vi "algo.get.state.vi"(11 "algo.data.in":T1={"next.state"=enum."Wait.for.Command", "saved.state"=enum."Wait.for.Command", "scratch"={"i"=0, "n"=0, "start.addr"=0, "first.call?"=FALSE, "j"=0, "o"=0, "k"=0, "p"=0, "just.write"=FALSE, "orderId "=0, "dir"=0}, "mode"=enum."Get.Symbol", "cmd.mem.watchlist"={"read.request"=FALSE, "read.addr"=0, "read.ready"=FALSE, "val.watchlist.read"={"symbol"=0, "buy.start.addr"=0, "buy.size"=0, "buy.slots"=0, "sell.start.addr"=0, "sell.size"=0, "sell.slots"=0, "min.ask"=0, "max.bid"=0}, "write.request"=FALSE, "write.addr"=0, "val.watchlist.write"={"symbol"=0, "buy.start.addr"=0, "buy.size"=0, "buy.slots"=0, "sell.start.addr"=0, "sell.size"=0, "sell.slots"=0, "min.ask"=0, "max.bid"=0}}, "cmd.mem.orders"={"read.addr"=0, "read.request"=FALSE, "read.ready"=FALSE, "write.addr"=0, "write.request"=FALSE, "read.data"={"OrderId"=0, "Price"=0, "Quantity"=0}, "write.data"={"OrderId"=0, "Price"=0, "Quantity"=0}}, "cmd.state"={"write.to.state"=FALSE, "val.state"=[0, 0, 0, 0]}, "cmd.debug"={"write.to.debug"=FALSE, "val.debug"=[0, 0]}, "stats"={"min.ask"=0, "max.bid"=0, "price"=0, "quantity"=0, "execution"=FALSE}, "orderbook.command"={"type"=enum."AddOrder", "side"=0, "orderId "=0, "quantity"=0, "symbol"=0, "price"=0, "executed.qty"=0, "canceled.qty"=0, "remaining.qty"=0, "seconds"=0, "nanoseconds"=0, "Add"=FALSE, "Edit"=FALSE, "Remove"=FALSE}, "time"={"last"=0, "since"=0}, "watchlist.size"=0, "active.watchlist"={"item"={"symbol"=0, "buy.start.addr"=0, "buy.size"=0, "buy.slots"=0, "sell.start.addr"=0, "sell.size"=0, "sell.slots"=0, "min.ask"=0, "max.bid"=0}, "index"=0}, "active.order"={"buy"=FALSE, "sell"=FALSE, "addr"=0, "size"=0, "slots"=0, "index"=0}} {"active.watchlist"."item"."symbol" format="%.0x"; "cmd.mem.orders"."write.data"."OrderId" format="%.0x"; "cmd.mem.orders"."read.data"."OrderId" format="%.0x"; "cmd.mem.watchlist"."val.watchlist.write"."symbol" format="%.0x"; "cmd.mem.watchlist"."val.watchlist.read"."symbol" format="%.0x"}) -> (3 "algo.data.out":T1={"next.state"=enum."Wait.for.Command", "saved.state"=enum."Wait.for.Command", "scratch"={"i"=0, "n"=0, "start.addr"=0, "first.call?"=FALSE, "j"=0, "o"=0, "k"=0, "p"=0, "just.write"=FALSE, "orderId "=0, "dir"=0}, "mode"=enum."Get.Symbol", "cmd.mem.watchlist"={"read.request"=FALSE, "read.addr"=0, "read.ready"=FALSE, "val.watchlist.read"={"symbol"=0, "buy.start.addr"=0, "buy.size"=0, "buy.slots"=0, "sell.start.addr"=0, "sell.size"=0, "sell.slots"=0, "min.ask"=0, "max.bid"=0}, "write.request"=FALSE, "write.addr"=0, "val.watchlist.write"={"symbol"=0, "buy.start.addr"=0, "buy.size"=0, "buy.slots"=0, "sell.start.addr"=0, "sell.size"=0, "sell.slots"=0, "min.ask"=0, "max.bid"=0}}, "cmd.mem.orders"={"read.addr"=0, "read.request"=FALSE, "read.ready"=FALSE, "write.addr"=0, "write.request"=FALSE, "read.data"={"OrderId"=0, "Price"=0, "Quantity"=0}, "write.data"={"OrderId"=0, "Price"=0, "Quantity"=0}}, "cmd.state"={"write.to.state"=FALSE, "val.state"=[0, 0, 0, 0]}, "cmd.debug"={"write.to.debug"=FALSE, "val.debug"=[0, 0]}, "stats"={"min.ask"=0, "max.bid"=0, "price"=0, "quantity"=0, "execution"=FALSE}, "orderbook.command"={"type"=enum."AddOrder", "side"=0, "orderId "=0, "quantity"=0, "symbol"=0, "price"=0, "executed.qty"=0, "canceled.qty"=0, "remaining.qty"=0, "seconds"=0, "nanoseconds"=0, "Add"=FALSE, "Edit"=FALSE, "Remove"=FALSE}, "time"={"last"=0, "since"=0}, "watchlist.size"=0, "active.watchlist"={"item"={"symbol"=0, "buy.start.addr"=0, "buy.size"=0, "buy.slots"=0, "sell.start.addr"=0, "sell.size"=0, "sell.slots"=0, "min.ask"=0, "max.bid"=0}, "index"=0}, "active.order"={"buy"=FALSE, "sell"=FALSE, "addr"=0, "size"=0, "slots"=0, "index"=0}} {"active.watchlist"."item"."symbol" format="%.0x"; "cmd.mem.orders"."write.data"."OrderId" format="%.0x"; "cmd.mem.orders"."read.data"."OrderId" format="%.0x"; "cmd.mem.watchlist"."val.watchlist.write"."symbol" format="%.0x"; "cmd.mem.watchlist"."val.watchlist.read"."symbol" format="%.0x"})   [LabVIEW 2020]
uses:
  types/algo.mode.ctl
  types/algo.states.ctl
  types/algo.scratch.ctl
  types/algo.val.watchlist.ctl
  types/algo.cmd.mem.watchlist.ctl
  types/algo.cmd.mem.orders.ctl
  types/algo.val.state.ctl
  types/algo.cmd.state.ctl
  types/algo.val.debug.ctl
  types/algo.cmd.debug.ctl
  types/algo.stats.ctl
  common/orderbook.command.type.ctl
  common/orderbook.command.ctl
  types/algo.time.ctl
  algo.data.ctl
  types/algo.val.order.ctl
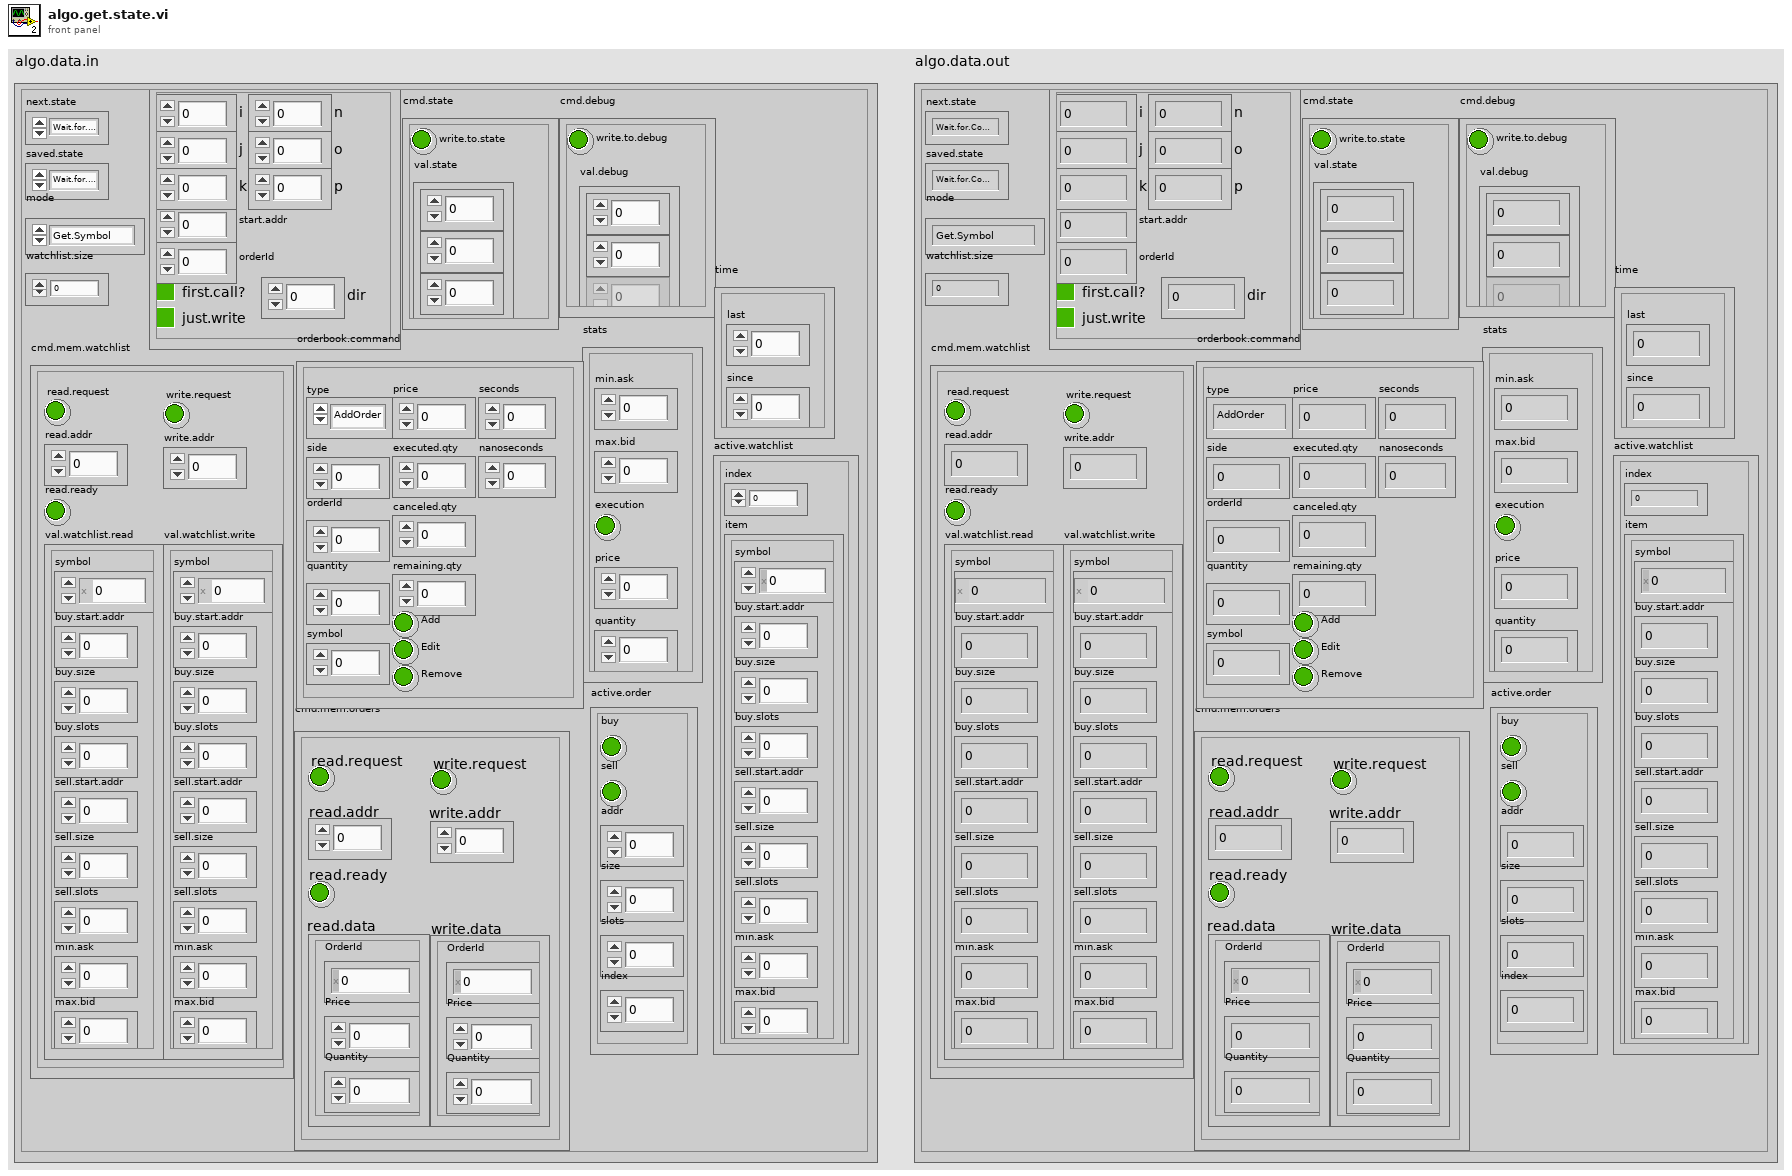
[diagram p1: front panel]
types:
  T1 = typedef "algo.data.ctl" = cluster{"next.state":T2, "saved.state":T2, "scratch":T3, "mode":T4, "cmd.mem.watchlist":T5, "cmd.mem.orders":T7, "cmd.state":T9, "cmd.debug":T11, "stats":T13, "orderbook.command":T14, "time":T16, "watchlist.size":u64, "active.watchlist":cluster{"item":T6, "index":u64}, "active.order":cluster{"buy":bool, "sell":bool, "addr":i16, "size":i16, "slots":i16, "index":i16}}
  T2 = typedef "algo.states.ctl" = enum16{"Noop", "Reset", "Configuration", "Debug", "Get.State", "Wait.for.Command", "Process.Command"}
  T3 = typedef "algo.scratch.ctl" = cluster{"i":u64, "n":u64, "start.addr":u16, "first.call?":bool, "j":u64, "o":u64, "k":u64, "p":u64, "just.write":bool, "orderId ":u64, "dir":i8}
  T4 = typedef "algo.mode.ctl" = enum16{"watchlist.iter", "order.buy.iter", "order.sell.iter", "Get.Symbol", "Search", "Shift"}
  T5 = typedef "algo.cmd.mem.watchlist.ctl" = cluster{"read.request":bool, "read.addr":u16, "read.ready":bool, "val.watchlist.read":T6, "write.request":bool, "write.addr":u16, "val.watchlist.write":T6}
  T6 = typedef "algo.val.watchlist.ctl" = cluster{"symbol":u64, "buy.start.addr":u16, "buy.size":u16, "buy.slots":u16, "sell.start.addr":u16, "sell.size":u16, "sell.slots":u16, "min.ask":u64, "max.bid":u64}
  T7 = typedef "algo.cmd.mem.orders.ctl" = cluster{"read.addr":u16, "read.request":bool, "read.ready":bool, "write.addr":u16, "write.request":bool, "read.data":T8, "write.data":T8}
  T8 = typedef "algo.val.order.ctl" = cluster{"OrderId":u64, "Price":u64, "Quantity":u32}
  T9 = typedef "algo.cmd.state.ctl" = cluster{"write.to.state":bool, "val.state":T10}
  T10 = typedef "algo.val.state.ctl" = u64[]
  T11 = typedef "algo.cmd.debug.ctl" = cluster{"write.to.debug":bool, "val.debug":T12}
  T12 = typedef "algo.val.debug.ctl" = u64[]
  T13 = typedef "algo.stats.ctl" = cluster{"min.ask":u32, "max.bid":u32, "price":u32, "quantity":u32, "execution":bool}
  T14 = typedef "orderbook.command.ctl" = cluster{"type":T15, "side":u8, "orderId ":u64, "quantity":u32, "symbol":u64, "price":u64, "executed.qty":u32, "canceled.qty":u32, "remaining.qty":u32, "seconds":u64, "nanoseconds":u64, "Add":bool, "Edit":bool, "Remove":bool}
  T15 = typedef "orderbook.command.type.ctl" = enum8{"Time", "AddOrder", "OrderExecuted", "OrderExecutedAtPrice", "ReduceSize", "ModifyOrder", "DeleteOrder", "Get.Everything", "Get.All.Orders", "Get.Top"}
  T16 = typedef "algo.time.ctl" = cluster{"last":u32, "since":u32}
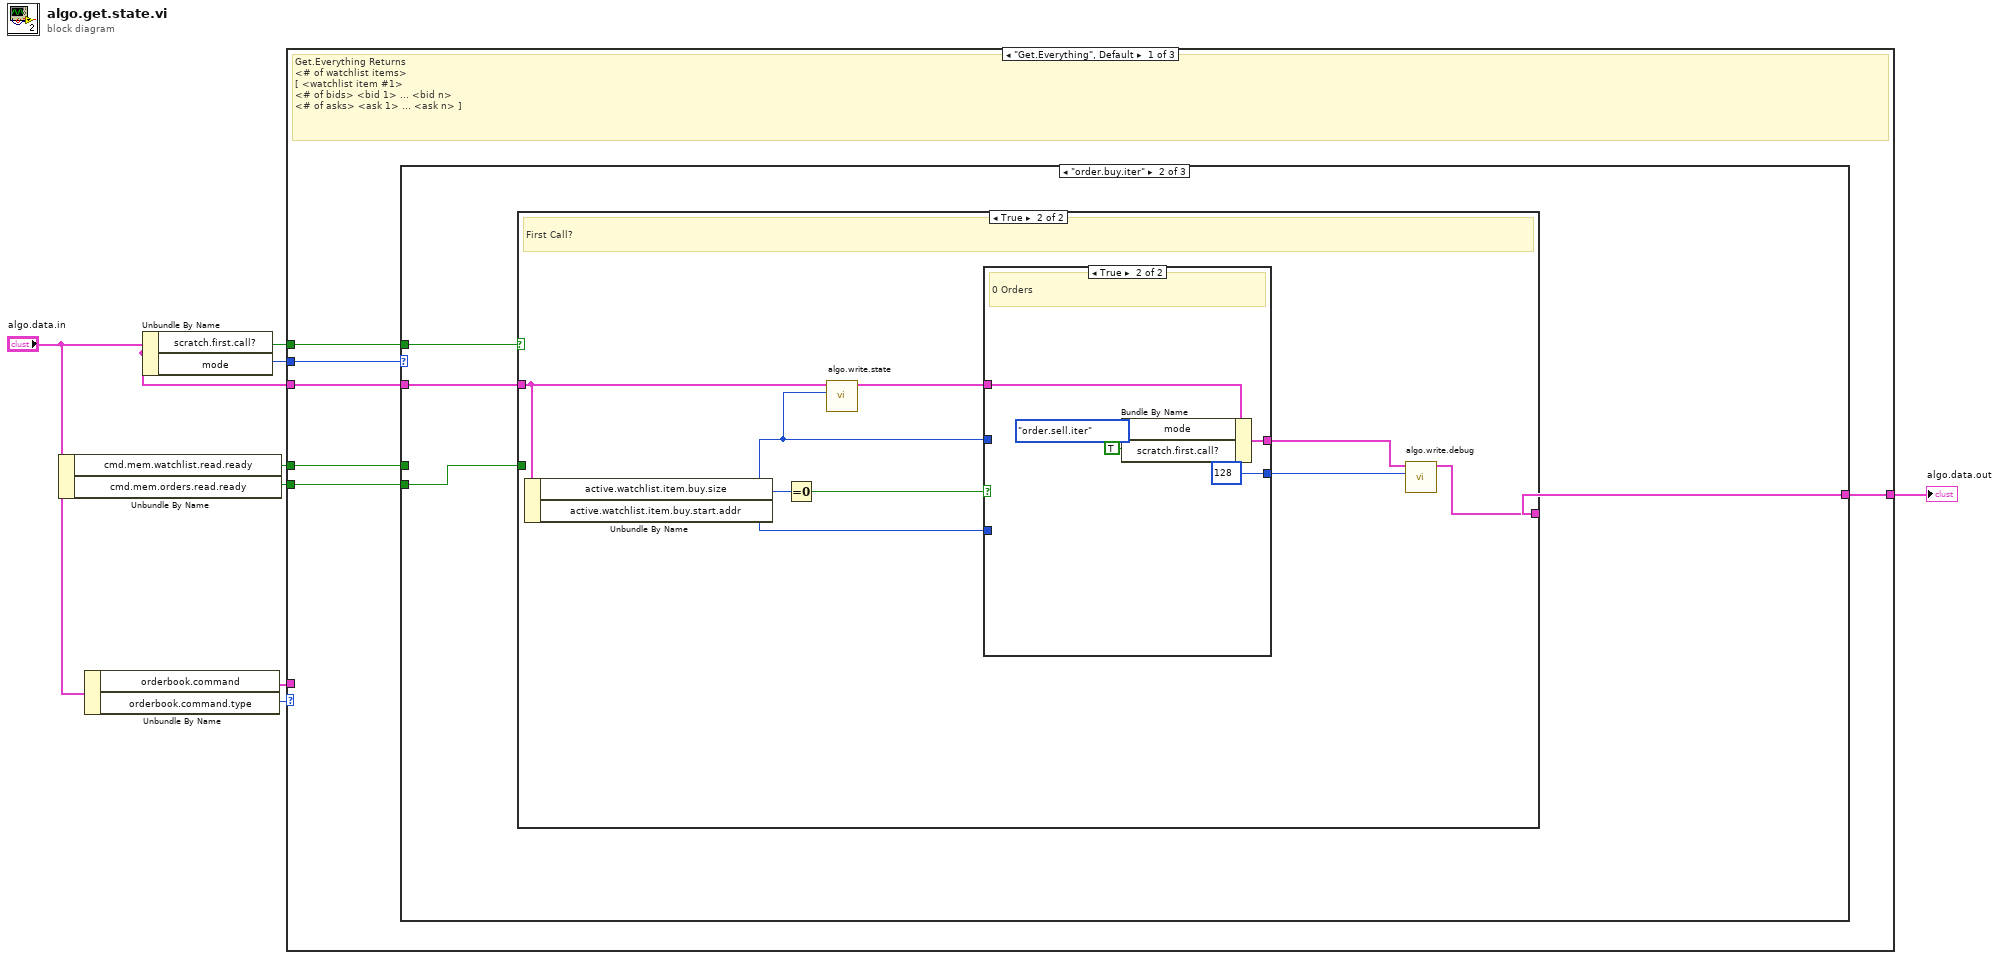
[diagram p0: block diagram]
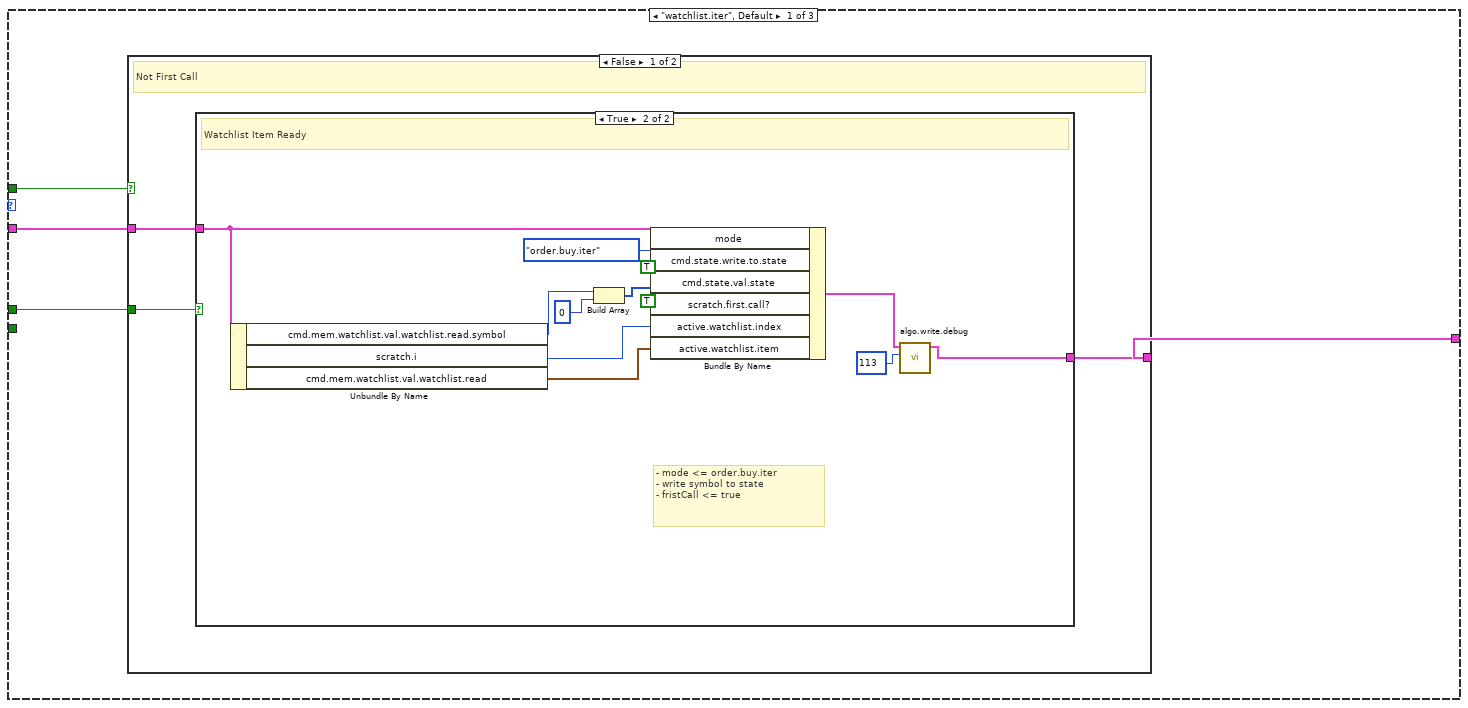
[diagram p2: hidden frame]
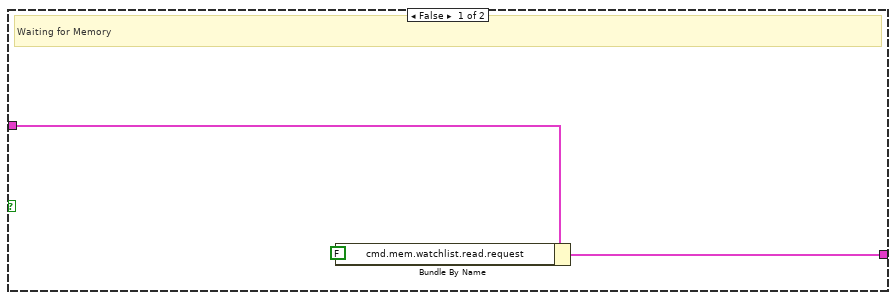
[diagram p3: hidden frame]
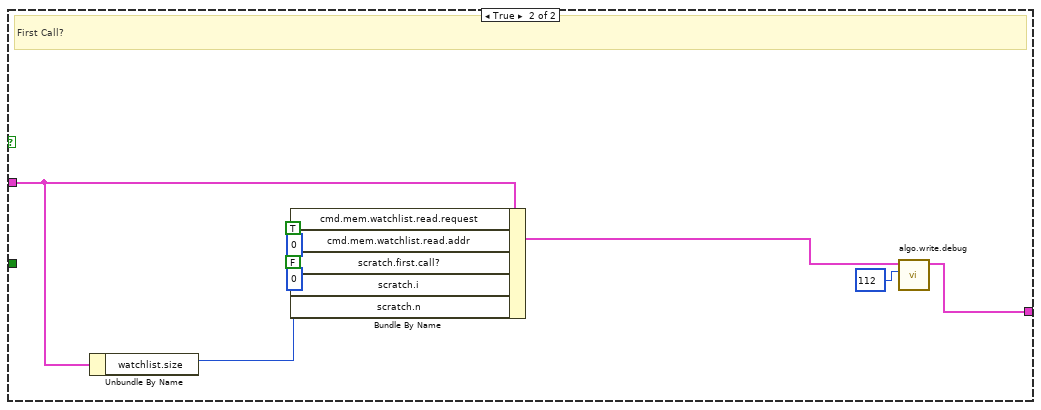
[diagram p4: hidden frame]
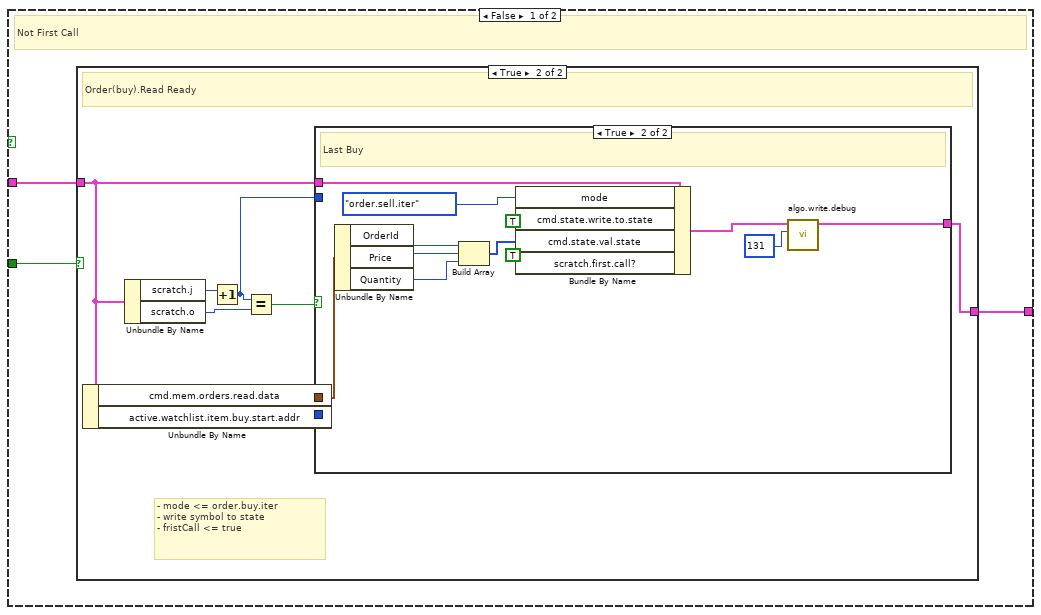
[diagram p5: hidden frame]
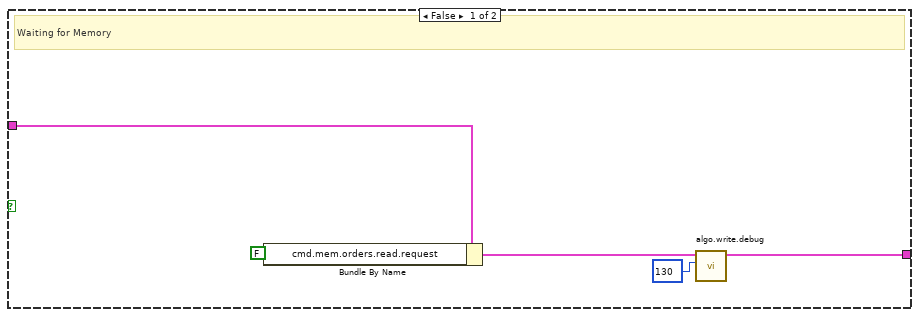
[diagram p6: hidden frame]
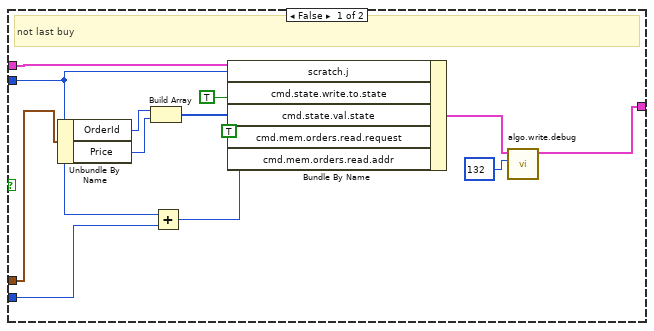
[diagram p7: hidden frame]
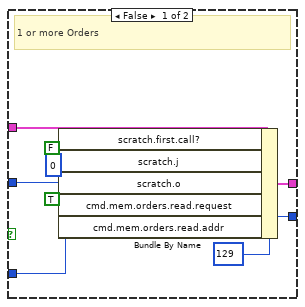
[diagram p8: hidden frame]
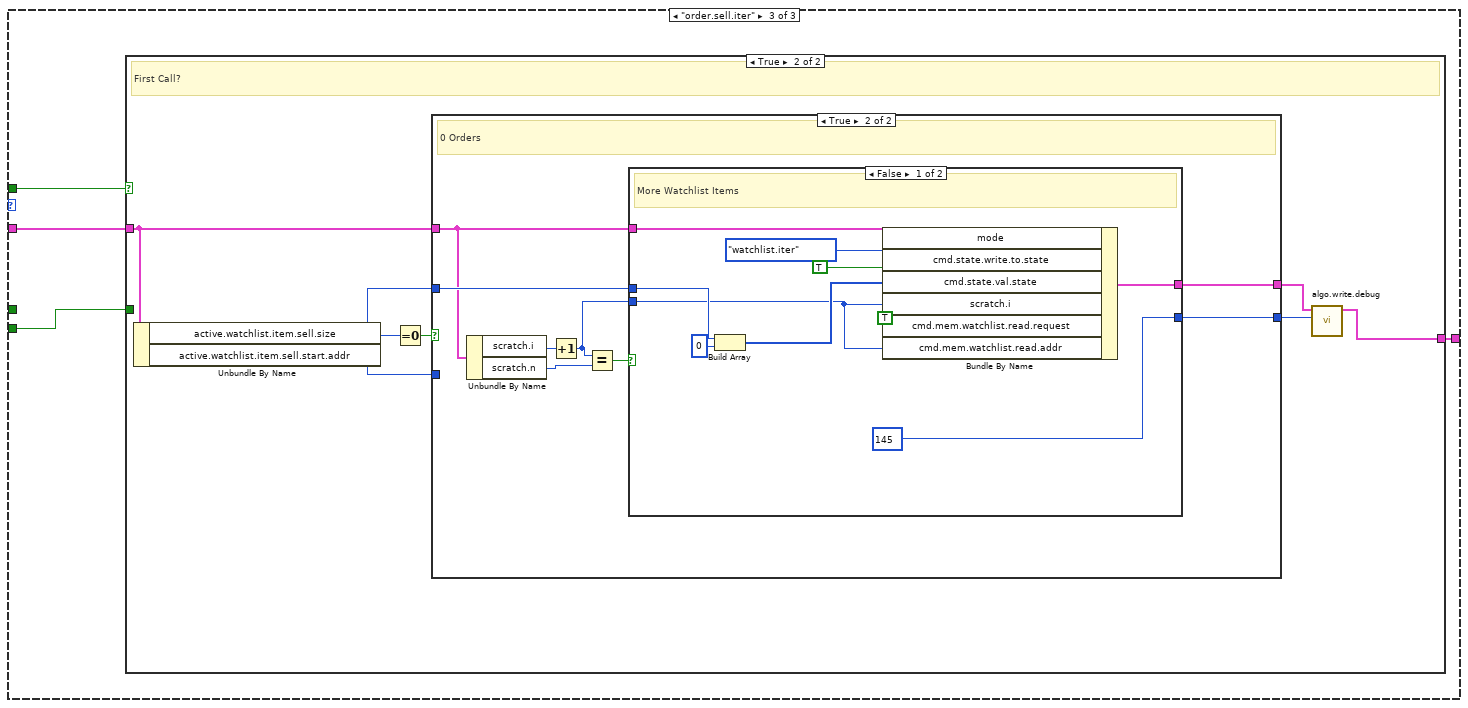
[diagram p9: hidden frame]
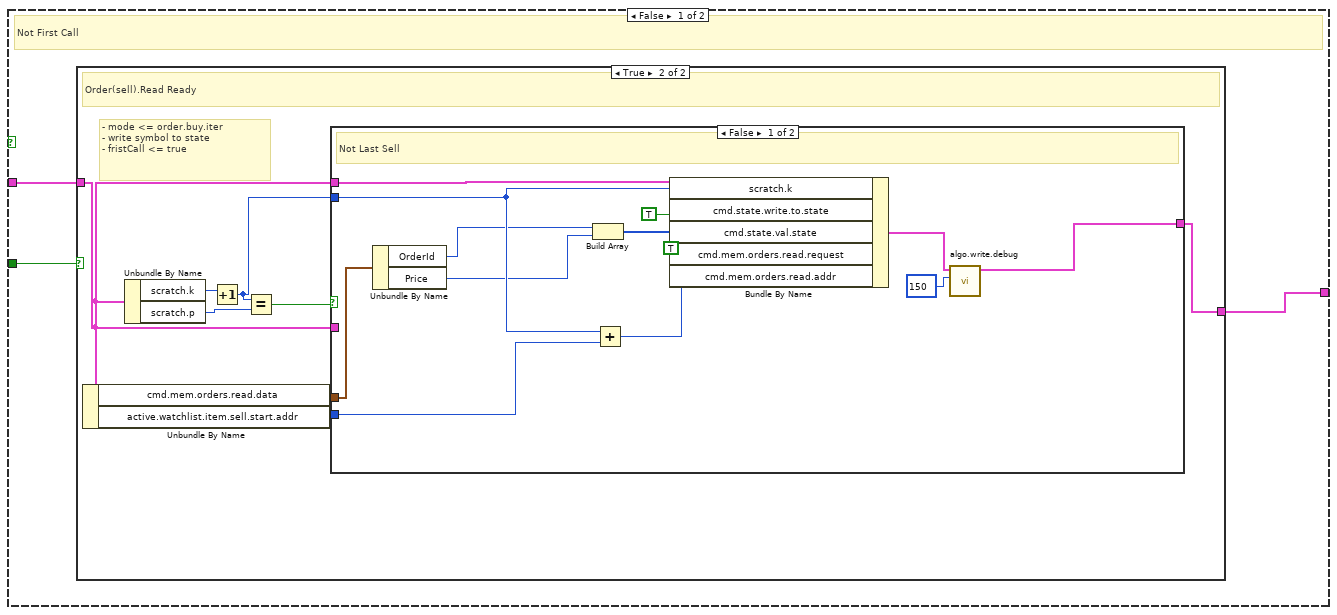
[diagram p10: hidden frame]
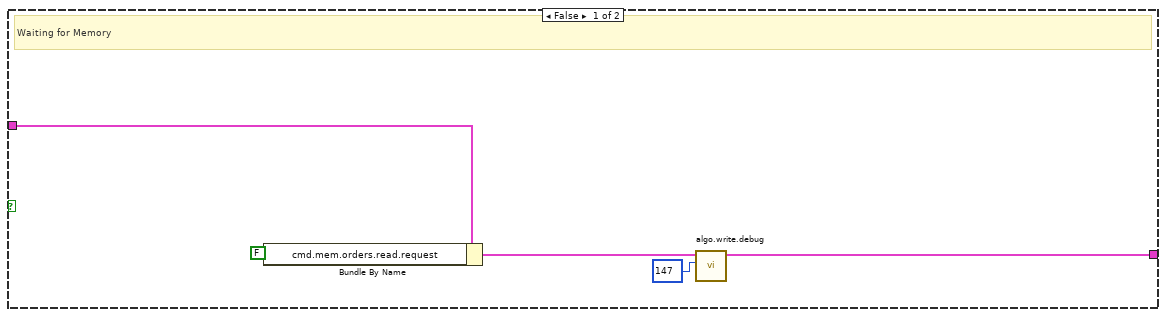
[diagram p11: hidden frame]
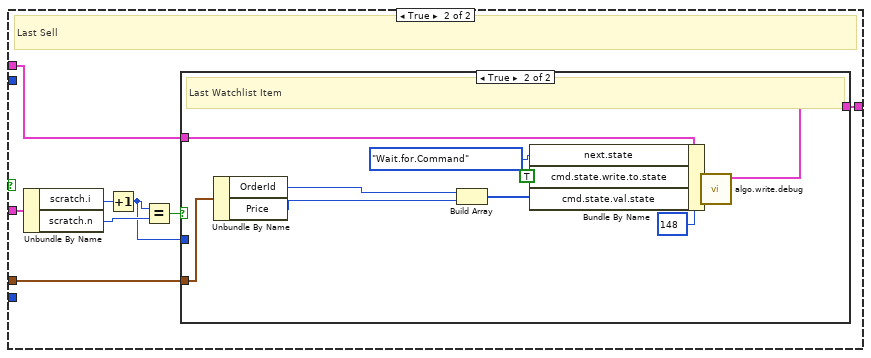
[diagram p12: hidden frame]
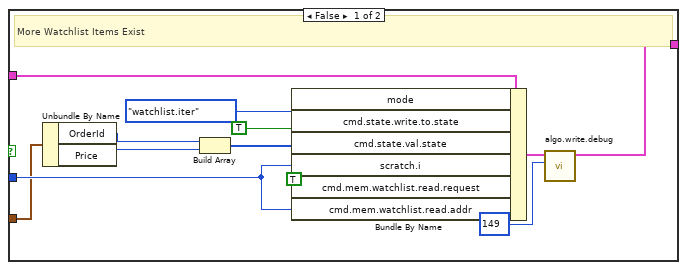
[diagram p13: hidden frame]
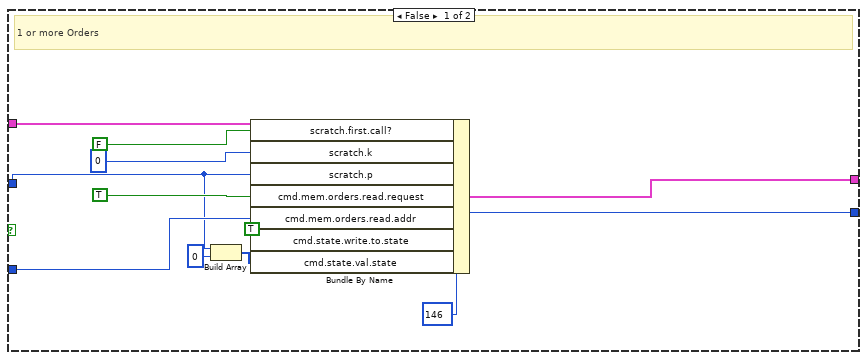
[diagram p14: hidden frame]
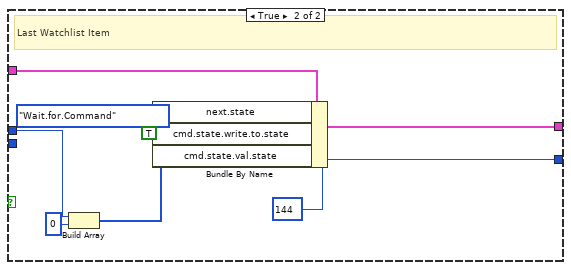
[diagram p15: hidden frame]
diagram:
  n1 = Unbundle By Name("algo.data.in") -> ("cmd.mem.watchlist.read.ready"=w3:bool, "cmd.mem.orders.read.ready"=w1:bool)
  n2 = Unbundle By Name("algo.data.in") -> ("orderbook.command"=w6:T14, "orderbook.command.type"=w5:T15)
  n3 = Unbundle By Name("algo.data.in") -> ("scratch.first.call?"=w7:bool, "mode"=w2:T4)
  n4 = case shown="\"Get.Everything\", Default" w5 {
    tunnel: [w12 w219 w220] -> w8
    tunnel: w7 -> [w14 _ _]
    tunnel: "algo.data.in" -> [w13 w219 w220]
    tunnel: w6 -> [_ _ _]
    tunnel: w3 -> [w11 _ _]
    tunnel: w2 -> [w10 _ _]
    tunnel: w1 -> [w9 _ _]
    frame "Get.Everything", Default {
      # "Get.Everything Returns \n<# of watchlist items>\n[ <watchlist item #1>\n<# of bids> <bid 1> ... <bid n>\n<# of asks> <ask 1> ... <ask n> ]"
      n5 = case shown="\"order.buy.iter\"" w10 {
        tunnel: w14 -> [w18 w46 w112]
        tunnel: w13 -> [w17 w49 w115]
        tunnel: [w16 w47 w113] -> w12
        tunnel: w11 -> [w15 _ _]
        tunnel: w9 -> [_ w48 w114]
        frame "watchlist.iter", Default {
          n6 = case shown="False" w18 {
            tunnel: w17 -> [w21 w38]
            tunnel: [w20 w45] -> w16
            tunnel: w15 -> [w19 _]
            frame False {
              # "Not First Call"
              n7 = case shown="True" w19 {
                tunnel: w21 -> [w24 w34]
                tunnel: [w23 w25] -> w20
                frame False {
                  # "Waiting for Memory"
                  n8 = Bundle By Name(cluster=w24, "cmd.mem.watchlist.read.request"=FALSE) -> (w23:T1)
                }
                frame True {
                  # "- mode <= order.buy.iter\n- write symbol to state\n- fristCall <= true"
                  # "Watchlist Item Ready"
                  n9 = Unbundle By Name(w34) -> ("cmd.mem.watchlist.val.watchlist.read.symbol"=w33:u64, "scratch.i"=w29:u64, "cmd.mem.watchlist.val.watchlist.read"=w28:T6)
                  n10 = Build Array(w33, u64 0 ("element")) -> (w31:u64[])
                  n11 = Bundle By Name(cluster=w34, "mode"=algo.mode."order.buy.iter", "cmd.state.write.to.state"=TRUE, "cmd.state.val.state"=w31, "scratch.first.call?"=TRUE, "active.watchlist.index"=w29, "active.watchlist.item"=w28) -> (w26:T1)
                  n12 = call "algo.write.debug.vi"("dbg.val.1"=u64 113 ("Dbg.Val.1"), "algo.data.in"=w26) -> ("algo.data.out"=w25:T1)  [unwired: 9 in]
                }
              }
            }
            frame True {
              # "First Call?"
              n13 = Unbundle By Name(w38) -> ("watchlist.size"=w37:u64)
              n14 = Bundle By Name(cluster=w38, "cmd.mem.watchlist.read.request"=TRUE, "cmd.mem.watchlist.read.addr"=u16 0, "scratch.first.call?"=FALSE, "scratch.i"=u64 0, "scratch.n"=w37) -> (w40:T1)
              n15 = call "algo.write.debug.vi"("dbg.val.1"=u64 112 ("Dbg.Val.1"), "algo.data.in"=w40) -> ("algo.data.out"=w45:T1)  [unwired: 9 in]
            }
          }
        }
        frame "order.buy.iter" {
          n16 = case shown="True" w46 {
            tunnel: w49 -> [w52 w92]
            tunnel: [w51 w98] -> w47
            tunnel: w48 -> [w50 _]
            frame False {
              # "Not First Call"
              n17 = case shown="True" w50 {
                tunnel: w52 -> [w57 w62]
                tunnel: [w53 w65] -> w51
                frame False {
                  # "Waiting for Memory"
                  n18 = Bundle By Name(cluster=w57, "cmd.mem.orders.read.request"=FALSE ("cmd.mem.watchlist.read.request")) -> (w54:T1)
                  n19 = call "algo.write.debug.vi"("dbg.val.1"=u64 130 ("Dbg.Val.1"), "algo.data.in"=w54) -> ("algo.data.out"=w53:T1)  [unwired: 9 in]
                }
                frame True {
                  # "- mode <= order.buy.iter\n- write symbol to state\n- fristCall <= true"
                  # "Order(buy).Read Ready"
                  n20 = Unbundle By Name(w62) -> ("cmd.mem.orders.read.data"=w60:T8, "active.watchlist.item.buy.start.addr"=w58:u16)
                  n21 = Unbundle By Name(w62) -> ("scratch.j"=w63:u64, "scratch.o"=w64:u64)
                  n22 = Increment(x=w63) -> (x+1=w59:u64)
                  n23 = Equal?(x=w59, y=w64) -> (x = y?=w61:bool)
                  n24 = case shown="True" w61 {
                    tunnel: w62 -> [w78 w88]
                    tunnel: [w76 w83] -> w65
                    tunnel: w60 -> [w68 w82]
                    tunnel: w59 -> [w71 _]
                    tunnel: w58 -> [w72 _]
                    frame False {
                      # "not last buy"
                      n25 = Unbundle By Name(w68) -> ("OrderId"=w67:u64, "Price"=w66:u64)
                      n26 = Build Array(w67, w66) -> (w73:u64[])
                      n27 = Add(x=w71, y=w72) -> (x+y=w70:u64)
                      n28 = Bundle By Name(cluster=w78, "scratch.j"=w71, "cmd.state.write.to.state"=TRUE, "cmd.state.val.state"=w73, "cmd.mem.orders.read.request"=TRUE, "cmd.mem.orders.read.addr"=w70) -> (w75:T1)
                      n29 = call "algo.write.debug.vi"("dbg.val.1"=u64 132 ("Dbg.Val.1"), "algo.data.in"=w75) -> ("algo.data.out"=w76:T1)  [unwired: 9 in]
                    }
                    frame True {
                      # "Last Buy"
                      n30 = Unbundle By Name(w82) -> ("OrderId"=w81:u64, "Price"=w80:u64, "Quantity"=w79:u32)
                      n31 = Build Array(w81, w80, w79) -> (w87:u64[])
                      n32 = Bundle By Name(cluster=w88, "mode"=algo.mode."order.sell.iter", "cmd.state.write.to.state"=TRUE, "cmd.state.val.state"=w87, "scratch.first.call?"=TRUE) -> (w84:T1)
                      n33 = call "algo.write.debug.vi"("dbg.val.1"=u64 131 ("Dbg.Val.1"), "algo.data.in"=w84) -> ("algo.data.out"=w83:T1)  [unwired: 9 in]
                    }
                  }
                }
              }
            }
            frame True {
              # "First Call?"
              n34 = Unbundle By Name(w92) -> ("active.watchlist.item.buy.size"=w93:u16, "active.watchlist.item.buy.start.addr"=w95:u16)
              n35 = Equal To 0?(x=w93) -> (x = 0?=w96:bool)
              n36 = call "algo.write.state.vi"("state.val.1"=w93, "algo.data.in"=w92) -> ("algo.data.out"=w91:T1)  [unwired: 9 in]
              n37 = case shown="True" w96 {
                tunnel: [w106 w111] -> w97
                tunnel: w91 -> [w99 w110]
                tunnel: w95 -> [w104 _]
                tunnel: w93 -> [w101 _]
                tunnel: [u64 129 ("Dbg.Val.1") u64 128 ("Dbg.Val.1")] -> w94
                frame False {
                  # "1 or more Orders"
                  n38 = Bundle By Name(cluster=w99, "scratch.first.call?"=FALSE, "scratch.j"=u64 0, "scratch.o"=w101, "cmd.mem.orders.read.request"=TRUE, "cmd.mem.orders.read.addr"=w104) -> (w106:T1)
                }
                frame True {
                  # "0 Orders"
                  n39 = Bundle By Name(cluster=w110, "mode"=algo.mode."order.sell.iter", "scratch.first.call?"=TRUE) -> (w111:T1)
                }
              }
              n40 = call "algo.write.debug.vi"("dbg.val.1"=w94, "algo.data.in"=w97) -> ("algo.data.out"=w98:T1)  [unwired: 9 in]
            }
          }
        }
        frame "order.sell.iter" {
          n41 = case shown="True" w112 {
            tunnel: w115 -> [w118 w179]
            tunnel: [w117 w181] -> w113
            tunnel: w114 -> [w116 _]
            frame False {
              # "Not First Call"
              n42 = case shown="True" w116 {
                tunnel: w118 -> [w123 w124]
                tunnel: [w119 w131] -> w117
                frame False {
                  # "Waiting for Memory"
                  n43 = Bundle By Name(cluster=w123, "cmd.mem.orders.read.request"=FALSE ("cmd.mem.watchlist.read.request")) -> (w120:T1)
                  n44 = call "algo.write.debug.vi"("dbg.val.1"=u64 147 ("Dbg.Val.1"), "algo.data.in"=w120) -> ("algo.data.out"=w119:T1)  [unwired: 9 in]
                }
                frame True {
                  # "- mode <= order.buy.iter\n- write symbol to state\n- fristCall <= true"
                  # "Order(sell).Read Ready"
                  n45 = Unbundle By Name(w124) -> ("cmd.mem.orders.read.data"=w127:T8, "active.watchlist.item.sell.start.addr"=w125:u16)
                  n46 = Unbundle By Name(w124) -> ("scratch.k"=w129:u64, "scratch.p"=w130:u64)
                  n47 = Increment(x=w129) -> (x+1=w126:u64)
                  n48 = Equal?(x=w126, y=w130) -> (x = y?=w128:bool)
                  n49 = case shown="False" w128 {
                    tunnel: w124 -> [w144 w152]
                    tunnel: [w142 w150] -> w131
                    tunnel: w127 -> [w134 w151]
                    tunnel: w126 -> [w137 _]
                    tunnel: w125 -> [w138 _]
                    tunnel: w124 -> [_ w147]
                    frame False {
                      # "Not Last Sell"
                      n50 = Unbundle By Name(w134) -> ("OrderId"=w132:u64, "Price"=w133:u64)
                      n51 = Build Array(w132, w133) -> (w139:u64[])
                      n52 = Add(x=w137, y=w138) -> (x+y=w136:u64)
                      n53 = Bundle By Name(cluster=w144, "scratch.k"=w137, "cmd.state.write.to.state"=TRUE, "cmd.state.val.state"=w139, "cmd.mem.orders.read.request"=TRUE, "cmd.mem.orders.read.addr"=w136) -> (w141:T1)
                      n54 = call "algo.write.debug.vi"("dbg.val.1"=u64 150 ("Dbg.Val.1"), "algo.data.in"=w141) -> ("algo.data.out"=w142:T1)  [unwired: 9 in]
                    }
                    frame True {
                      # "Last Sell"
                      n55 = Unbundle By Name(w147) -> ("scratch.i"=w149:u64, "scratch.n"=w148:u64)
                      n56 = Increment(x=w149) -> (x+1=w145:u64)
                      n57 = Equal?(x=w145, y=w148) -> (x = y?=w146:bool)
                      n58 = case shown="True" w146 {
                        tunnel: w152 -> [w164 w173]
                        tunnel: w151 -> [w155 w167]
                        tunnel: [w156 w169] -> w150
                        tunnel: w145 -> [w159 _]
                        frame False {
                          # "More Watchlist Items Exist"
                          n59 = Unbundle By Name(w155) -> ("OrderId"=w154:u64, "Price"=w153:u64)
                          n60 = Build Array(w154, w153) -> (w162:u64[])
                          n61 = Bundle By Name(cluster=w164, "mode"=algo.mode."watchlist.iter", "cmd.state.write.to.state"=TRUE, "cmd.state.val.state"=w162, "scratch.i"=w159, "cmd.mem.watchlist.read.request"=TRUE, "cmd.mem.watchlist.read.addr"=w159) -> (w158:T1)
                          n62 = call "algo.write.debug.vi"("dbg.val.1"=u64 149 ("Dbg.Val.1"), "algo.data.in"=w158) -> ("algo.data.out"=w156:T1)  [unwired: 9 in]
                        }
                        frame True {
                          # "Last Watchlist Item"
                          n63 = Unbundle By Name(w167) -> ("OrderId"=w166:u64, "Price"=w165:u64)
                          n64 = Build Array(w166, w165) -> (w172:u64[])
                          n65 = Bundle By Name(cluster=w173, "next.state"=algo.states."Wait.for.Command", "cmd.state.write.to.state"=TRUE, "cmd.state.val.state"=w172) -> (w170:T1)
                          n66 = call "algo.write.debug.vi"("dbg.val.1"=u64 148 ("Dbg.Val.1"), "algo.data.in"=w170) -> ("algo.data.out"=w169:T1)  [unwired: 9 in]
                        }
                      }
                    }
                  }
                }
              }
            }
            frame True {
              # "First Call?"
              n67 = Unbundle By Name(w179) -> ("active.watchlist.item.sell.size"=w176:u16, "active.watchlist.item.sell.start.addr"=w177:u16)
              n68 = Equal To 0?(x=w176) -> (x = 0?=w178:bool)
              n69 = case shown="True" w178 {
                tunnel: [w191 w200] -> w180
                tunnel: w179 -> [w192 w197]
                tunnel: w177 -> [w189 _]
                tunnel: w176 -> [w182 w198]
                tunnel: [u64 146 ("Dbg.Val.1") w199] -> w175
                frame False {
                  # "1 or more Orders"
                  n70 = Build Array(w182, u16 0 ("element")) -> (w183:u16[])
                  n71 = Bundle By Name(cluster=w192, "scratch.first.call?"=FALSE, "scratch.k"=u64 0 ("scratch.j"), "scratch.p"=w182, "cmd.mem.orders.read.request"=TRUE, "cmd.mem.orders.read.addr"=w189, "cmd.state.write.to.state"=TRUE, "cmd.state.val.state"=w183) -> (w191:T1)
                }
                frame True {
                  # "0 Orders"
                  n72 = Unbundle By Name(w197) -> ("scratch.i"=w195:u64, "scratch.n"=w196:u64)
                  n73 = Increment(x=w195) -> (x+1=w193:u64)
                  n74 = Equal?(x=w193, y=w196) -> (x = y?=w194:bool)
                  n75 = case shown="False" w194 {
                    tunnel: [w203 w218] -> w200
                    tunnel: w197 -> [w209 w217]
                    tunnel: [u64 145 ("Dbg.Val.1") u64 144 ("Dbg.Val.1")] -> w199
                    tunnel: w198 -> [w207 w212]
                    tunnel: w193 -> [w202 _]
                    frame False {
                      # "More Watchlist Items"
                      n76 = Build Array(w207, u16 0 ("element")) -> (w205:u16[])
                      n77 = Bundle By Name(cluster=w209, "mode"=algo.mode."watchlist.iter", "cmd.state.write.to.state"=TRUE, "cmd.state.val.state"=w205, "scratch.i"=w202, "cmd.mem.watchlist.read.request"=TRUE, "cmd.mem.watchlist.read.addr"=w202) -> (w203:T1)
                    }
                    frame True {
                      # "Last Watchlist Item"
                      n78 = Build Array(w212, u16 0 ("element")) -> (w215:u16[])
                      n79 = Bundle By Name(cluster=w217, "next.state"=algo.states."Wait.for.Command", "cmd.state.write.to.state"=TRUE, "cmd.state.val.state"=w215) -> (w218:T1)
                    }
                  }
                }
              }
              n80 = call "algo.write.debug.vi"("dbg.val.1"=w175, "algo.data.in"=w180) -> ("algo.data.out"=w181:T1)  [unwired: 9 in]
            }
          }
        }
      }
    }
    frame "Get.All.Orders" {
    }
    frame "Get.Top" {
    }
  }
  "algo.data.out" <- w8
